vi "Periodic Tasks.vi"() -> ()   [LabVIEW 2011]
doc: "This VI runs in parallel to other tasks. It can contain as many user-defined periodic loops as you need. These can carry out PID or other sorts of timed response."
uses:
  <vilib>/Rock Robotics/SystemInterfaces/Utilities/FPGA_UtilitiesLED State.ctl
  <vilib>/Rock Robotics/SystemInterfaces/Utilities/FPGA_UtilitiesLED Source.ctl
  Robot Global Data.vi
  <vilib>/Rock Robotics/WPI/Relay/WPI_RelayValue.ctl
panel:
  out "Rate 3":dbl
  out "error out 4":errorcluster
  out "Direction 3":bool
  out "Distance 3":dbl
  out "Distance 2":dbl
  out "Direction 2":bool
  out "error out 3":errorcluster
  out "Rate 2":dbl
  out "Rate":dbl
  out "error out 2":errorcluster
  out "I2C":bool
  out "Angular Rate":dbl
  out "Angle":dbl
  out "Direction":bool
  out "Distance":dbl
  # "Speed to move to home"
  # "Target Tracking"
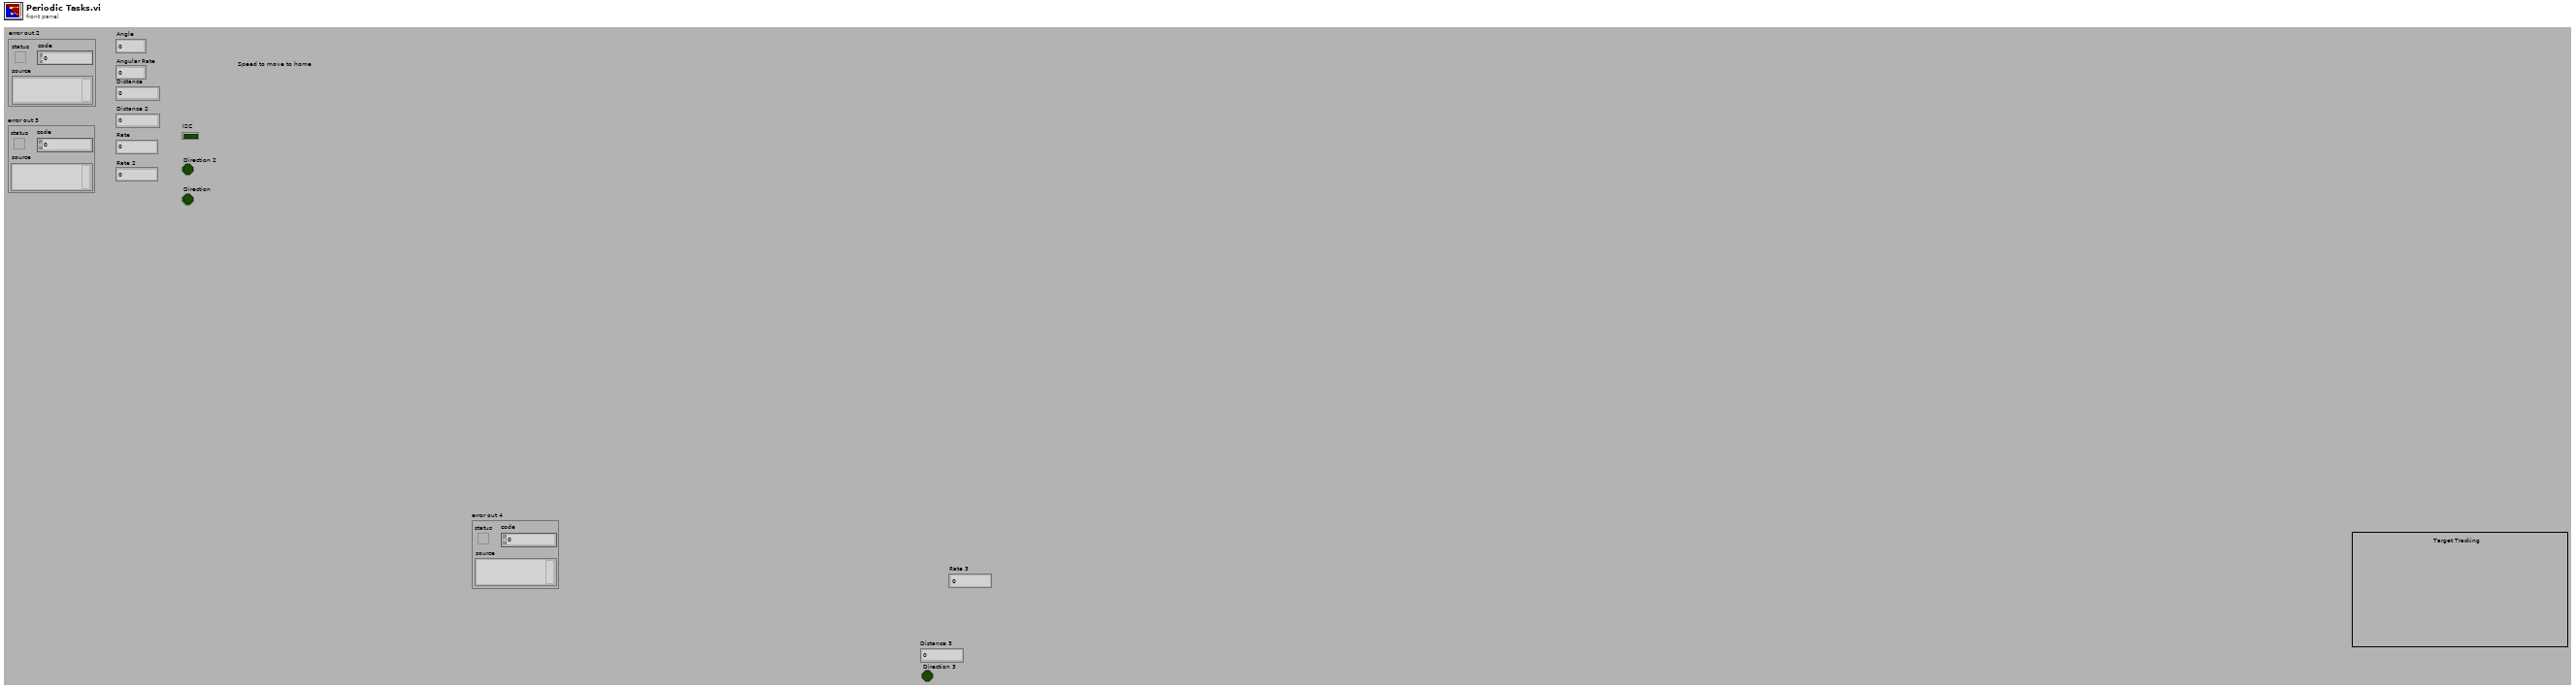
[diagram p1: front panel]
types:
  T1 = typedef "WPI_RelayValue.ctl" = enum16{"Off", "On", "Forward", "Reverse"}
  T2 = typedef "WPI_AnalogChannelDevRef.ctl" = cluster{"DevStatus":errorcluster, "Analog Module":T3, "Analog Channel":T4}
  T3 = typedef "FPGA_TypedefAnalogModule.ctl" = enum16{"Analog Module 1", "Analog Module 2"}
  T4 = typedef "FPGA_AIChannel.ctl" = enum8{"AI 1", "AI 2", "AI 3", "AI 4", "AI 5", "AI 6", "AI 7", "AI 8", "Invalid"}
  T5 = typedef "WPI_EncoderDevRef.ctl" = cluster{"DevStatus":errorcluster, "EncoderIndex":T6, "CounterIndex":T7, "DistancePerCount":dbl, "Decoding Type":T8}
  T6 = typedef "FPGA_EncoderIdx.ctl" = enum8{"Enc 0", "Enc 1", "Enc 2", "Enc 3", "Invalid"}
  T7 = typedef "FPGA_CounterCtrSystemIndex.ctl" = enum8{"Ctr 0", "Ctr 1", "Ctr 2", "Ctr 3", "Ctr 4", "Ctr 5", "Ctr 6", "Ctr 7", "Invalid"}
  T8 = typedef "WPI_EncoderType.ctl" = enum16{"1x", "2x", "4x"}
  T9 = typedef "WPI_RelayDevRef.ctl" = cluster{"DevStatus":errorcluster, "Relay Channel":T10, "Digital Module":T11, "Relay Direction":T12}
  T10 = typedef "FPGA_DIORelayChannel.ctl" = enum8{"Relay 1", "Relay 2", "Relay 3", "Relay 4", "Relay 5", "Relay 6", "Relay 7", "Relay 8", "Invalid"}
  T11 = typedef "FPGA_TypedefDigitalModule.ctl" = enum16{"Digital Module 1", "Digital Module 2"}
  T12 = typedef "WPI_RelayDirection.ctl" = enum16{"Both directions", "Forward only", "Reverse only"}
  T13 = typedef "WPI_GyroDevRef.ctl" = cluster{"DevStatus":errorcluster, "Analog Module":T3, "Analog Channel":T4, "Offset":dbl, "Gain (VoltsPerDegree/Second)":dbl}
  T14 = cluster{"Driver Station Digital Output (1-8)[0]":bool, "Driver Station Digital Output (1-8)[1]":bool, "Driver Station Digital Output (1-8)[2]":bool, "Driver Station Digital Output (1-8)[3]":bool, "Driver Station Digital Output (1-8)[4]":bool, "Driver Station Digital Output (1-8)[5]":bool, "Driver Station Digital Output (1-8)[6]":bool, "Driver Station Digital Output (1-8)[7]":bool, "Driver Station Digital Output (1-8)[8]":bool}
  T15 = typedef "FPGA_UtilitiesLED State.ctl" = enum16{"Off", "On", "Toggle"}
  T16 = typedef "FPGA_UtilitiesLED Source.ctl" = enum16{"User LED", "FPGA LED"}
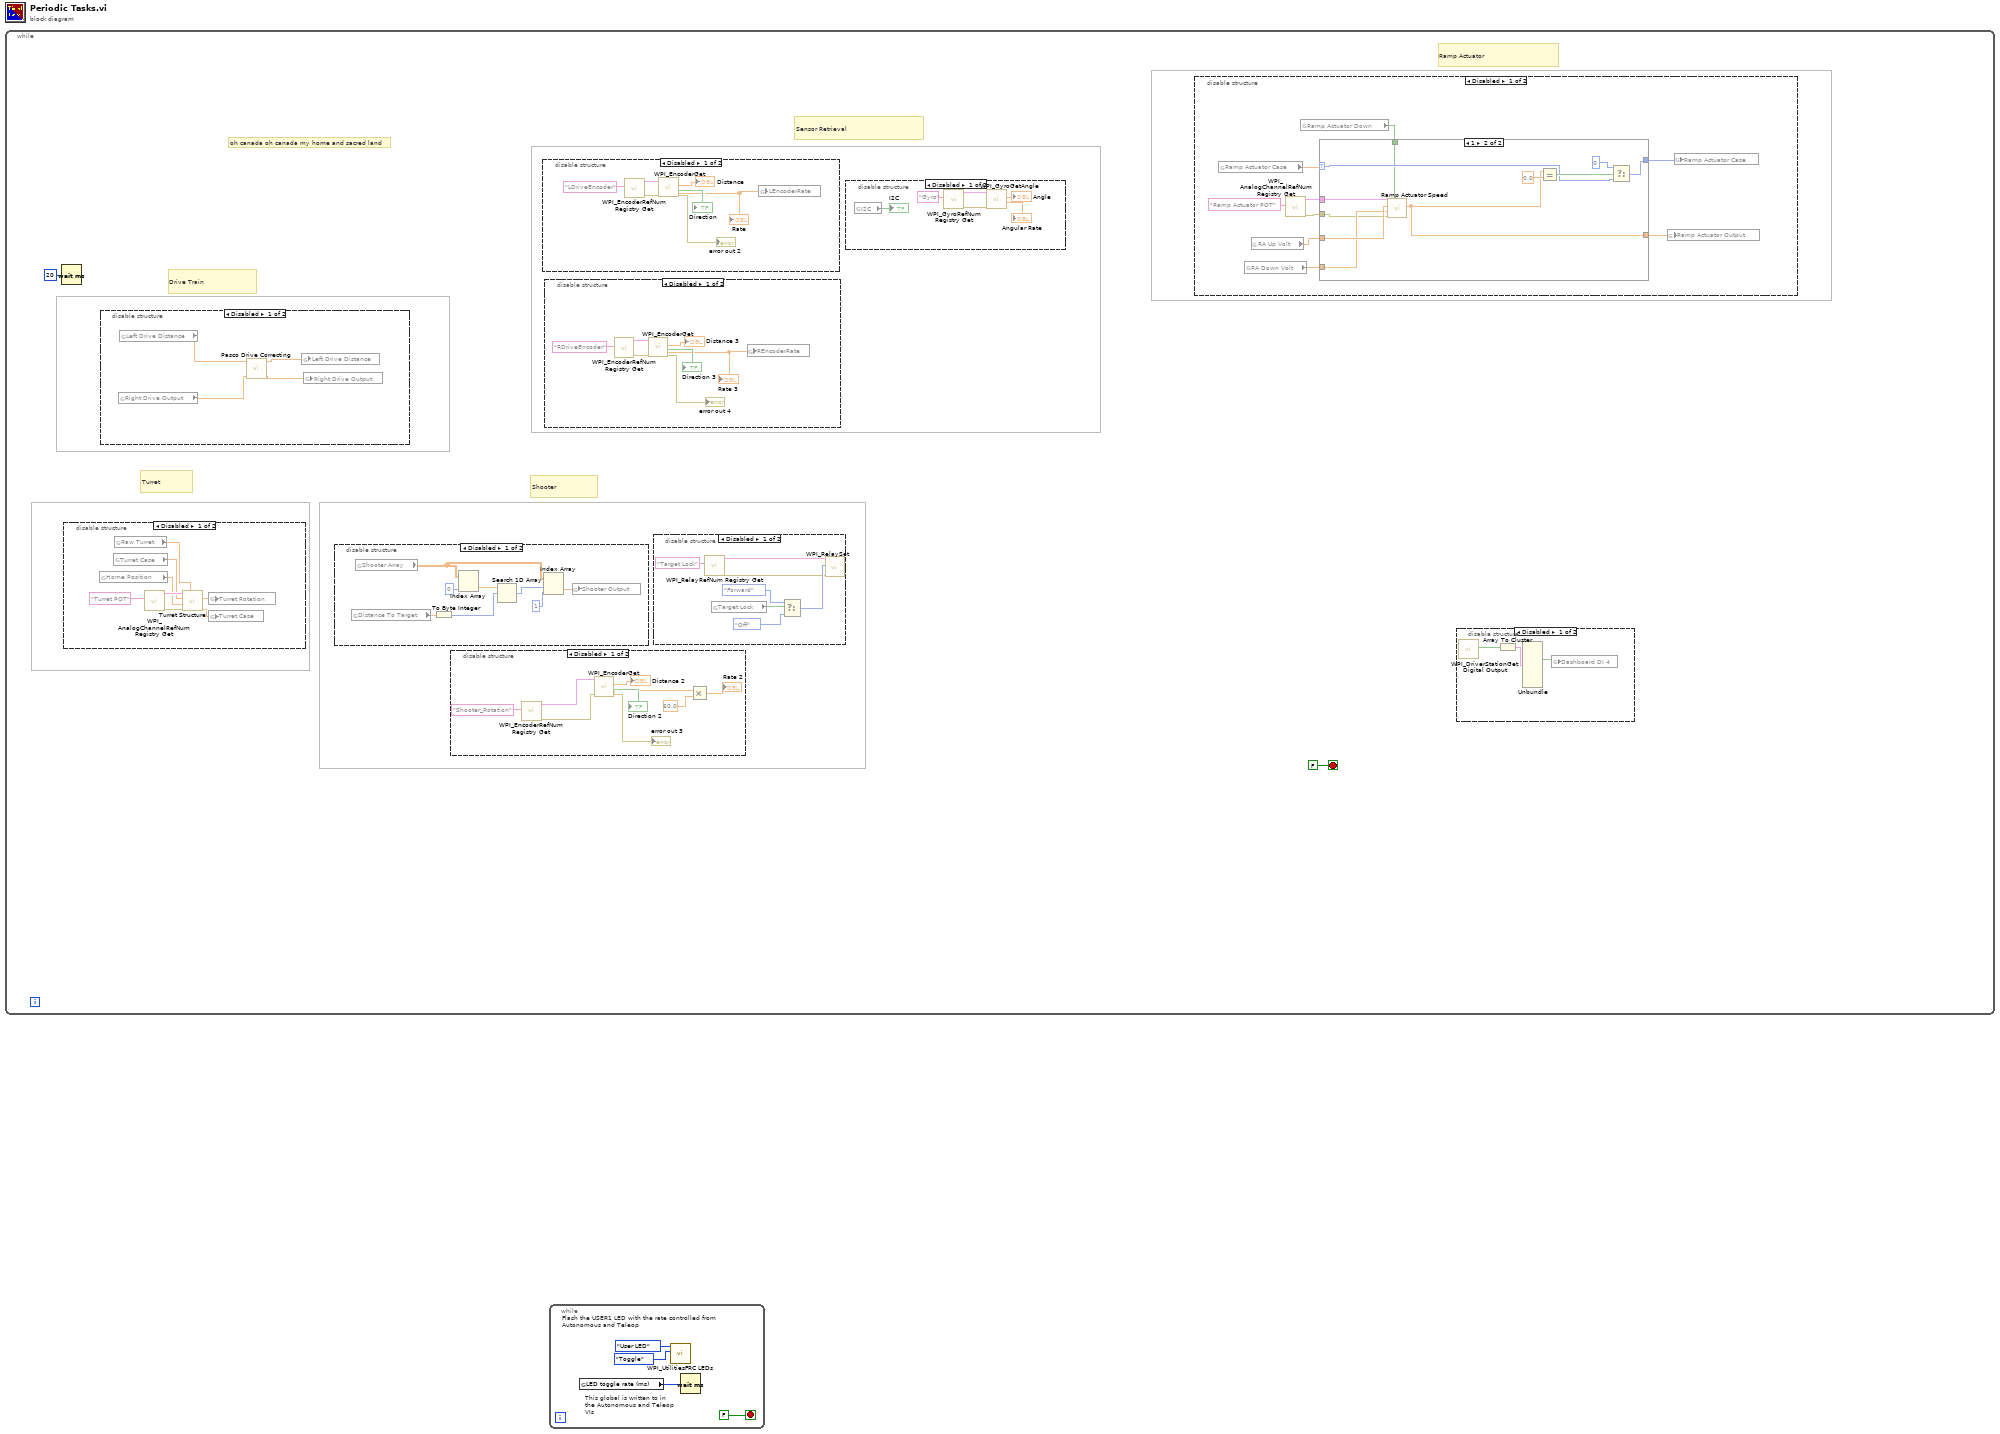
[diagram p0: block diagram]
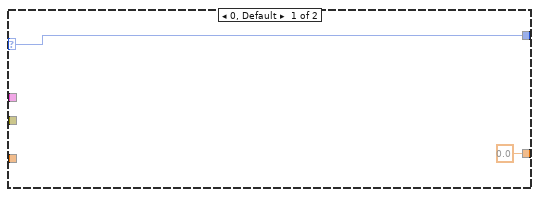
[diagram p3: hidden frame]
diagram:
  n1 = while {
    stop <- FALSE stop-if-true
    # "oh canada oh canada my home and sacred land"
    # "Shooter"
    # "Sensor Retrieval"
    # "Turret"
    # "Drive Train"
    # "Ramp Actuator"
    n2 = Wait (ms)(milliseconds to wait=u32 20) -> ()  [unwired: 1 out]
    n3 = disable-structure shown="Disabled" {
      frame Disabled {
        n4 = global read "Robot Global Data.vi" "Home Position"() -> (w35:dbl)
        n5 = global read "Robot Global Data.vi" "Turret Case"() -> (w36:dbl)
        n6 = global read "Robot Global Data.vi" "Raw Turret"() -> (w34:dbl)
        n7 = call <vilib>:"WPI_AnalogChannelRefNum Registry Get.vi"("refnum name"="Turret POT") -> ("error out"=w37:errorcluster, "AIDeviceRef"=w38:T2)  [unwired: 9 in]
        n8 = call "Turret Structure.vi"("Raw Turret"=w34, "error in (no error)"=w37, "Home postion"=w35, "Turret Case"=w36, "AIDeviceRef"=w38) -> ("Turret Case Output"=w32:dbl, "Turret Output"=w33:dbl)  [unwired: 5 in]
        n9 = global write "Robot Global Data.vi" "Turret Rotation"(w33) -> ()
        n10 = global write "Robot Global Data.vi" "Turret Case"(w32) -> ()
      }
      frame Enabled {
      }
    }
    n11 = disable-structure shown="Disabled" {
      frame Disabled {
        n12 = global read "Robot Global Data.vi" "Right Drive Output"() -> (w50:dbl)
        n13 = global read "Robot Global Data.vi" "Left Drive Distance"() -> (w51:dbl)
        n14 = call "Pasco Drive Correcting.vi"("RightDriveOutput"=w50, "LeftDriveOutput"=w51) -> ("RightDriveOutput"=w48:dbl, "LeftDriveOutput"=w49:dbl)  [unwired: 8 in]
        n15 = global write "Robot Global Data.vi" "Left Drive Distance"(w49) -> ()
        n16 = global write "Robot Global Data.vi" "Right Drive Output"(w48) -> ()
      }
      frame Enabled {
      }
    }
    n17 = disable-structure shown="Disabled" {
      frame Disabled {
        n18 = global read "Robot Global Data.vi" "Distance To Target"() -> (w45:dbl)
        n19 = global read "Robot Global Data.vi" "Shooter Array"() -> (w43:dbl[][])
        n20 = To Byte Integer(number=w45) -> (8bit integer=w44:i8)
        n21 = Index Array(array=w43, index (col)=0 ("disabled index (col)")) -> (element=w46:dbl[])  [unwired: 1 in]
        n22 = Search 1D Array(1D array=w46, element=w44) -> (index of element=w42:i32)  [unwired: 1 in]
        n23 = Index Array(array=w43, index (row)=w42, index (col)=1 ("disabled index (col)")) -> (element=w40:dbl)
        n24 = global write "Robot Global Data.vi" "Shooter Output"(w40) -> ()
      }
      frame Enabled {
      }
    }
    n25 = disable-structure shown="Disabled" {
      frame Disabled {
        n26 = call <vilib>:"WPI_EncoderRefNum Registry Get.vi"("refnum name"="Shooter_Rotation") -> ("error out"=w75:errorcluster, "EncoderDevRef"=w76:T5)  [unwired: 9 in]
        n27 = call <vilib>:"WPI_EncoderGet.vi"("error in (no error)"=w75, "EncoderDevRef"=w76) -> ("error out"=→"error out 3":errorcluster, "Direction"=→"Direction 2":bool, "Distance"=→"Distance 2":dbl, "Rate"=w79:dbl)  [unwired: 4 in, 2 out]
        n28 = Multiply(x=w79, y=60.0) -> (x*y=→"Rate 2":dbl)
      }
      frame Enabled {
      }
    }
    n29 = disable-structure shown="Disabled" {
      frame Disabled {
        n30 = call <vilib>:"WPI_EncoderRefNum Registry Get.vi"("refnum name"="LDriveEncoder") -> ("error out"=w66:errorcluster, "EncoderDevRef"=w65:T5)  [unwired: 9 in]
        n31 = call <vilib>:"WPI_EncoderGet.vi"("error in (no error)"=w66, "EncoderDevRef"=w65) -> ("error out"=→"error out 2":errorcluster, "Direction"=→"Direction":bool, "Distance"=→"Distance":dbl, "Rate"=w62:dbl)  [unwired: 4 in, 2 out]
        "Rate" <- w62
        n32 = global write "Robot Global Data.vi" "LEncoderRate"(w62) -> ()
      }
      frame Enabled {
      }
    }
    n33 = disable-structure shown="Disabled" {
      frame Disabled {
        n34 = call <vilib>:"WPI_EncoderRefNum Registry Get.vi"("refnum name"="RDriveEncoder") -> ("error out"=w59:errorcluster, "EncoderDevRef"=w58:T5)  [unwired: 9 in]
        n35 = call <vilib>:"WPI_EncoderGet.vi"("error in (no error)"=w59, "EncoderDevRef"=w58) -> ("error out"=→"error out 4":errorcluster, "Direction"=→"Direction 3":bool, "Distance"=→"Distance 3":dbl, "Rate"=w55:dbl)  [unwired: 4 in, 2 out]
        "Rate 3" <- w55
        n36 = global write "Robot Global Data.vi" "REncoderRate"(w55) -> ()
      }
      frame Enabled {
      }
    }
    n37 = disable-structure shown="Disabled" {
      frame Disabled {
        n38 = call <vilib>:"WPI_RelayRefNum Registry Get.vi"("refnum name"="Target Lock") -> ("error out"=w3:errorcluster, "RelayDevRef"=w4:T9)  [unwired: 9 in]
        n39 = global read "Robot Global Data.vi" "Target Lock"() -> (w9:bool)
        n40 = Select(t=WPI_RelayValue."Forward" ("RelayValue"), s=w9, f=WPI_RelayValue."Off" ("RelayValue")) -> (s? t:f=w6:T1)
        n41 = call <vilib>:"WPI_RelaySet.vi"("error in (no error)"=w3, "RelayValue"=w6, "RelayDevRef"=w4) -> ()  [unwired: 7 in, 2 out]
      }
      frame Enabled {
      }
    }
    n42 = disable-structure shown="Disabled" {
      frame Disabled {
        n43 = global read "Robot Global Data.vi" "I2C"() -> (→"I2C":bool)
        n44 = call <vilib>:"WPI_GyroRefNum Registry Get.vi"("refnum name"="Gyro") -> ("error out"=w73:errorcluster, "GyroDevRef"=w74:T13)  [unwired: 9 in]
        n45 = call <vilib>:"WPI_GyroGetAngle.vi"("error in (no error)"=w73, "GyroDevRef"=w74) -> ("Angular Rate"=→"Angular Rate":dbl, "Angle"=→"Angle":dbl)  [unwired: 6 in, 2 out]
      }
      frame Enabled {
      }
    }
    n46 = disable-structure shown="Disabled" {
      frame Disabled {
        n47 = global read "Robot Global Data.vi" "Ramp Actuator Case"() -> (w18:dbl)
        n48 = global read "Robot Global Data.vi" "RA Down Volt"() -> (w13:dbl)
        n49 = global read "Robot Global Data.vi" "RA Up Volt"() -> (w14:dbl)
        n50 = call <vilib>:"WPI_AnalogChannelRefNum Registry Get.vi"("refnum name"="Ramp Actuator POT") -> ("error out"=w11:errorcluster, "AIDeviceRef"=w12:T2)  [unwired: 9 in]
        n51 = global read "Robot Global Data.vi" "Ramp Actuator Down"() -> (w10:bool)
        n52 = case shown="1" w18 {
          selector: w18 -> [w20 w25]
          tunnel: [w20 w22] -> w17
          tunnel: [0.0 ("f") w23] -> w15
          tunnel: w14 -> [_ w31]
          tunnel: w13 -> [_ w30]
          tunnel: w12 -> [_ w29]
          tunnel: w11 -> [_ w28]
          tunnel: w10 -> [_ w21]
          frame 0, Default {
          }
          frame 1 {
            n53 = call "Ramp Actuator Speed.vi"("Up to Down"=w21, "error in (no error)"=w28, "RA Down Volt"=w30, "RA Up Volt"=w31, "AIDeviceRef"=w29) -> ("Ramp Actuator Ouput"=w23:dbl)  [unwired: 6 in]
            n54 = Equal?(x=w23, y=0.0) -> (x = y?=w26:bool)
            n55 = Select(t=0, s=w26, f=w25) -> (s? t:f=w22:i32)
          }
        }
        n56 = global write "Robot Global Data.vi" "Ramp Actuator Output"(w15) -> ()
        n57 = global write "Robot Global Data.vi" "Ramp Actuator Case"(w17) -> ()
      }
      frame Enabled {
      }
    }
    n58 = disable-structure shown="Disabled" {
      frame Disabled {
        n59 = call <vilib>:"WPI_DriverStationGet Digital Output.vi"() -> ("Driver Station Digital Output (1-8)"=w54:bool[])  [unwired: 10 in, 1 out]
        n60 = Array To Cluster(array=w54) -> (cluster=w53:T14)
        n61 = Unbundle(w53) -> ("Driver Station Digital Output (1-8)[3]"=w52:bool)  [unwired: 8 out]
        n62 = global write "Robot Global Data.vi" "Dashboard DI 4"(w52) -> ()
      }
      frame Enabled {
      }
    }
  }
  n63 = while {
    stop <- FALSE stop-if-true
    # "This global is written to in the Autonomous and Teleop VIs"
    # "Flash the USER1 LED with the rate controlled from Autonomous and Teleop"
    n64 = global read "Robot Global Data.vi" "LED toggle rate (ms)"() -> (w84:u32)
    n65 = call <vilib>:"WPI_UtilitiesFRC LEDs.vi"("State"=FPGA_UtilitiesLED_State."Toggle", "LED Type"=FPGA_UtilitiesLED_Source."User LED") -> ()  [unwired: 1 in, 9 out]
    n66 = Wait (ms)(milliseconds to wait=w84) -> ()  [unwired: 1 out]
  }
